vi "Teleop.vi"(11 "Call Context":T1) -> ()   [LabVIEW 2013]
doc: "This VI is called for each TeleOp packet received from the DS where the robot is not disabled. It is often used to read from the joysticks and update I/O or to update setpoints for timed control loops. It should complete and return within 20 milliseconds or it may miss DS packets."
uses:
  <vilib>/Rock Robotics/WPI/DriverStation/WPI_DriverStationDerivedRobotMode.ctl
  Robot Global Data.vi
  Controller 1.vi
  Controller 2.vi
panel:
  in  "Rotation Mult":dbl=0.7
  in  "Joystick Mult Slow":dbl=0.3
  in  "Joystick Mult":dbl=1.0
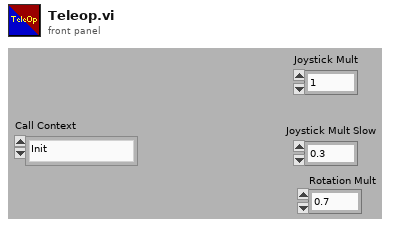
[diagram p1: front panel]
types:
  T1 = typedef "WPI_DriverStationDerivedRobotMode.ctl" = enum16{"Init", "Execute", "Stop"}
  T2 = cluster{"Axes":cluster{"LS X":dbl, "LS Y":dbl, "Triggers":dbl, "RS X":dbl, "RS Y":dbl}, "Buttons":cluster{"LT":bool, "RT":bool, "A":bool, "B":bool, "X":bool, "Y":bool, "LB":bool, "RB":bool, "Back":bool, "Start":bool, "LS":bool, "RS":bool}, "Buttons Just Pushed":cluster{"LT":bool, "RT":bool, "A":bool, "B":bool, "X":bool, "Y":bool, "LB":bool, "RB":bool, "Back":bool, "Start":bool, "LS":bool, "RS":bool}}
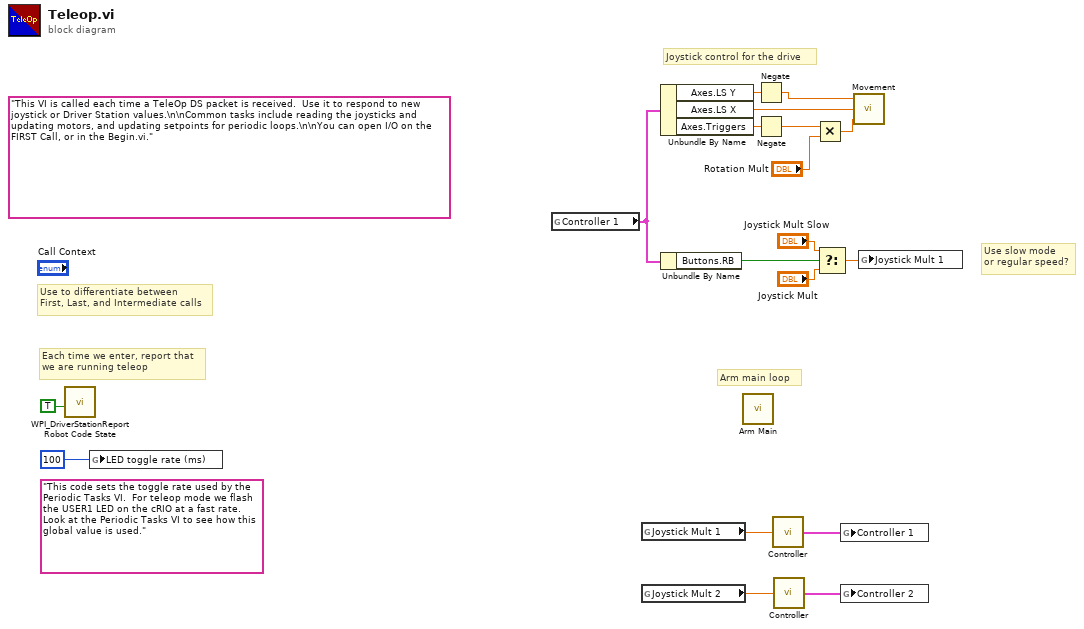
[diagram p0: block diagram]
diagram:
  (unwired) "This code sets the toggle rate used by the Periodic Tasks VI.  For teleop mode we flash the USER1 LED on the cRIO at a fast rate.  Look at the Periodic Tasks VI to see how this global value is used."
  (unwired) "This VI is called each time a TeleOp DS packet is received.  Use it to respond to new joystick or Driver Station values.\n\nCommon tasks include reading the joysticks and updating motors, and updating setpoints for periodic loops.\n\nYou can open I/O on the FIRST Call, or in the Begin.vi."
  # "Arm main loop"
  # "Joystick control for the drive"
  # "Use slow mode\nor regular speed?"
  # "Each time we enter, report that\nwe are running teleop"
  # "Use to differentiate between\nFirst, Last, and Intermediate calls"
  n1 = call <vilib>:"WPI_DriverStationReport Robot Code State.vi"("TeleOp"=TRUE ("Autonomous")) -> ()  [unwired: 10 in, 1 out]
  n2 = global write "Robot Global Data.vi" "LED toggle rate (ms)"(u32 100 ("LED ms toggle rate")) -> ()
  n3 = global read "Robot Global Data.vi" "Controller 1"() -> (w12:T2)
  n4 = global read "Robot Global Data.vi" "Joystick Mult 1"() -> (w6:dbl)
  n5 = global read "Robot Global Data.vi" "Joystick Mult 2"() -> (w7:dbl)
  n6 = Unbundle By Name(w12) -> ("Axes.LS Y"=w10:dbl, "Axes.LS X"=w9:dbl, "Axes.Triggers"=w8:dbl)
  n7 = Unbundle By Name(w12) -> ("Buttons.RB"=w11:bool)
  n8 = call "Arm Main.vi"() -> ()  [unwired: 1 out]
  n9 = Negate(x=w10) -> (-x=w14:dbl)
  n10 = Negate(x=w8) -> (-x=w3:dbl)
  n11 = call-poly "Controller.vi"("Joystick Multiplier"=w6) -> ("Values"=w5:T2)
  n12 = call-poly "Controller.vi"("Joystick Multiplier"=w7) -> ("Values"=w4:T2)
  n13 = Multiply(x=w3, y="Rotation Mult") -> (x*y=w2:dbl)
  n14 = Select(t="Joystick Mult Slow", s=w11, f="Joystick Mult") -> (s? t:f=w13:dbl)
  n15 = global write "Robot Global Data.vi" "Controller 1"(w5) -> ()
  n16 = global write "Robot Global Data.vi" "Controller 2"(w4) -> ()
  n17 = call "Movement.vi"("Rotational Speed"=w2, "Sideways Speed"=w9, "Forward Speed"=w14) -> ()
  n18 = global write "Robot Global Data.vi" "Joystick Mult 1"(w13) -> ()
